vi "Build data.vi"(1 "Hold":bool, 2 "Input":cluster{"Y":dbl[], "Y":dbl[]}[](array[cluster])) -> (0 "Output":cluster{"Y":dbl[], "Y":dbl[]}[](array[cluster]))   [LabVIEW 2020]
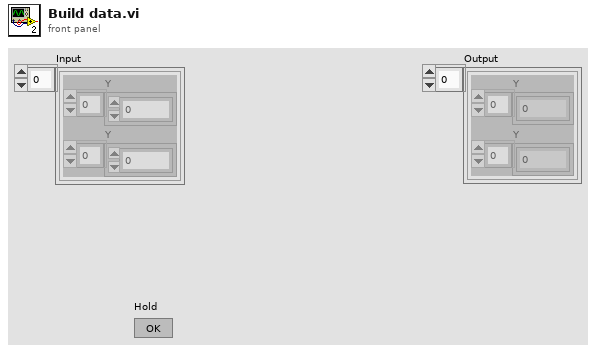
[diagram p1: front panel]
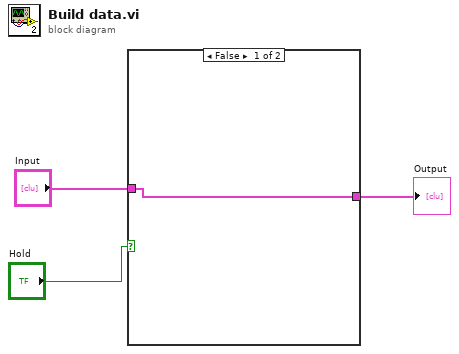
[diagram p0: block diagram]
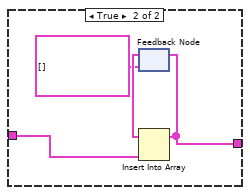
[diagram p2: hidden frame]
diagram:
  n1 = case shown="False" "Hold" {
    tunnel: "Input" -> [w4 w7]
    tunnel: [w4 w5] -> w2
    frame False {
    }
    frame True {
      n2 = feedback #1(cluster{"Y":dbl[], "Y":dbl[]}[] []) -> (w8:cluster{"Y":dbl[], "Y":dbl[]}[])
      n3 = Insert Into Array(array=w8, new element=w7) -> (w5:cluster{"Y":dbl[], "Y":dbl[]}[])  [unwired: 1 in]
      n4 = feedback-in #1(w5) -> ()
    }
  }
  "Output" <- w2
